vi "Get Limit Status.vi"(8 "error in (no error)":errorcluster {"code" format="%.0x"}, 10 "Device Number (1)":i32=1, 11 "VISA Resource Name":refnum<visa-resource-name>) -> (0 "error out":errorcluster {"code" format="%.0x"}, 2 "Status":T1(ring), 3 "VISA Resource Name Out":refnum<visa-resource-name>)   [LabVIEW 2020, in "Olympus IX BX Series.lvlib"]
doc: "Gets the status of the limit of the focusing unit movement."
uses:
  Olympus IX BX Series.lvlib
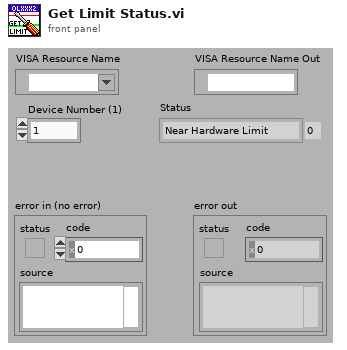
[diagram p1: front panel]
types:
  T1 = enum16{"Near Hardware Limit", "Near Software Limit", "Normal Range", "Far Software Limit", "Far Hardware Limit", "Anomalous Software Limit", "Unknown"}
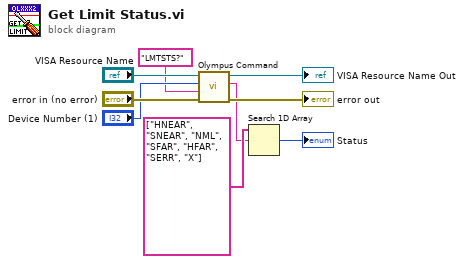
[diagram p0: block diagram]
diagram:
  n1 = call "Olympus Command.vi"("error in (no error)"="error in (no error)", "Command string"="LMTSTS?" ("format string"), "Device Number (1)"="Device Number (1)", "VISA Resource Name"="VISA Resource Name") -> ("error out"=→"error out":errorcluster, "Result"=w2:string, "VISA Resource Name Out"=→"VISA Resource Name Out":refnum<visa-resource-name>)  [unwired: 5 in]
  n2 = Search 1D Array(1D array=string[] ["HNEAR", "SNEAR", "NML", "SFAR", "HFAR", "SERR", "X"], element=w2) -> (index of element=→"Status":i32)  [unwired: 1 in]
